vi "7903 Port 5 Constructor.vi"(11 "aurora instance (0)":u8) -> (3 "aurora64b66b buffered":refnum<class "Aurora64b66b Buffered.lvclass">)   [LabVIEW 2023, in "PXIe-7903 Aurora Example.lvlib"]
uses:
  PXIe-7903 Aurora Example.lvlib
  Program Files/NI/LVAddons/niidl/1/instr.lib/_niInstr/Aurora64b66b/v1/Shared/Buffered/Link Mode.ctl
  Program Files/NI/LVAddons/niidl/1/instr.lib/_niInstr/Aurora64b66b/v1/Shared/niInstr Aurora64b66b v1 Shared.lvlib
  Program Files/NI/LVAddons/niidl/1/instr.lib/_niInstr/Aurora64b66b/v1/Shared/Basic/Endianness.ctl
  Program Files/NI/LVAddons/niidl/1/instr.lib/_niInstr/Aurora64b66b/v1/Shared/Basic/GT Type.ctl
  Program Files/NI/LVAddons/niidl/1/instr.lib/_niInstr/Aurora64b66b/v1/Shared/Basic/Aurora Config.ctl
  Program Files/NI/LVAddons/niidl/1/instr.lib/_niInstr/CLIP Adapters/v1/FPGA/AXI4-Lite/FXP32 Address - FXP32 Data/Public/CLIP Resources.ctl
  Program Files/NI/LVAddons/niidl/1/instr.lib/_niInstr/CLIP Adapters/v1/FPGA/AXI4-Lite/FXP32 Address - FXP32 Data/niInstr AXI4-Lite - FXP32 Address - FXP32 Data v1 FPGA.lvclass
  Program Files/NI/LVAddons/niidl/1/instr.lib/_niInstr/Aurora64b66b/v1/FPGA/Basic/Public/TypeDefs/CLIP Parameters.ctl
  Program Files/NI/LVAddons/niidl/1/instr.lib/_niInstr/Aurora64b66b/v1/FPGA/Basic/Aurora64b66b Basic.lvclass
  Program Files/NI/LVAddons/niidl/1/instr.lib/_niInstr/Aurora64b66b/v1/FPGA/Buffered/Aurora64b66b Buffered.lvclass
  Program Files/NI/LVAddons/niidl/1/instr.lib/_niInstr/Aurora64b66b/v1/FPGA/Basic/Public/TypeDefs/Tx Data CLIP IO.ctl
  Program Files/NI/LVAddons/niidl/1/instr.lib/_niInstr/Aurora64b66b/v1/FPGA/Basic/Public/TypeDefs/Rx Data CLIP IO.ctl
  Program Files/NI/LVAddons/niidl/1/instr.lib/_niInstr/Aurora64b66b/v1/FPGA/Basic/Public/TypeDefs/NFC CLIP IO.ctl
  Program Files/NI/LVAddons/niidl/1/instr.lib/_niInstr/Aurora64b66b/v1/FPGA/Basic/Public/TypeDefs/Link Status CLIP IO.ctl
  Program Files/NI/LVAddons/niidl/1/instr.lib/_niInstr/Aurora64b66b/v1/FPGA/Basic/Public/TypeDefs/Reset CLIP IO.ctl
  Program Files/NI/LVAddons/niidl/1/instr.lib/_niInstr/Aurora64b66b/v1/FPGA/Basic/Public/TypeDefs/CRC CLIP IO.ctl
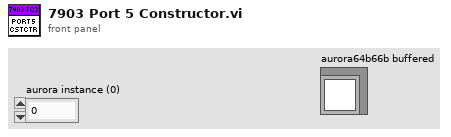
[diagram p1: front panel]
types:
  T1 = typedef "niInstr Aurora64b66b v1 FPGA.lvlib/Aurora64b66b Basic.lvclass/CLIP Parameters.ctl" = cluster{"crc clip io":T2, "reset clip io":T3, "link status clip io":T4, "nfc clip io":T5, "user clock":refnum<k21>, "rx data ":T6, "tx data":T7, "axi drp clip resources":T8, "axi control clip resources":T8}
  T2 = typedef "niInstr Aurora64b66b v1 FPGA.lvlib/Aurora64b66b Basic.lvclass/CRC CLIP IO.ctl" = cluster{"crc pass fail n":refnum<k21>, "crc valid":refnum<k21>}
  T3 = typedef "niInstr Aurora64b66b v1 FPGA.lvlib/Aurora64b66b Basic.lvclass/Reset CLIP IO.ctl" = cluster{"reset pb":refnum<k21>, "pma init":refnum<k21>, "link reset":refnum<k21>}
  T4 = typedef "niInstr Aurora64b66b v1 FPGA.lvlib/Aurora64b66b Basic.lvclass/Link Status CLIP IO.ctl" = cluster{"hard error":refnum<k21>, "soft error":refnum<k21>, "lane up 8":refnum<k21>, "channel up":refnum<k21>, "sys reset":refnum<k21>, "mmcm not locked":refnum<k21>, "lane up 4":refnum<k21>}
  T5 = typedef "niInstr Aurora64b66b v1 FPGA.lvlib/Aurora64b66b Basic.lvclass/NFC CLIP IO.ctl" = cluster{"s_axis_tvalid":refnum<k21>, "s_axis_tdata":refnum<k21>, "s_axis_tready":refnum<k21>}
  T6 = typedef "niInstr Aurora64b66b v1 FPGA.lvlib/Aurora64b66b Basic.lvclass/Rx Data CLIP IO.ctl" = cluster{"m_axis_tvalid":refnum<k21>, "m_axis_tdata0":refnum<k21>, "m_axis_tdata1":refnum<k21>, "m_axis_tdata 2":refnum<k21>, "m_axis_tdata 3":refnum<k21>, "m_axis_tdata4":refnum<k21>, "m_axis_tdata5":refnum<k21>, "m_axis_tdata6":refnum<k21>, "m_axis_tdata7":refnum<k21>, "m_axis_tlast":refnum<k21>, "m_axis_tkeep1":refnum<k21>, "m_axis_tkeep2":refnum<k21>, "m_axis_tkeep4":refnum<k21>, "m_axis_tkeep8":refnum<k21>}
  T7 = typedef "niInstr Aurora64b66b v1 FPGA.lvlib/Aurora64b66b Basic.lvclass/Tx Data CLIP IO.ctl" = cluster{"s_axis_tvalid":refnum<k21>, "s_axis_tdata0":refnum<k21>, "s_axis_tdata1":refnum<k21>, "s_axis_tdata2":refnum<k21>, "s_axis_tdata3":refnum<k21>, "s_axis_tdata4":refnum<k21>, "s_axis_tdata5":refnum<k21>, "s_axis_tdata6":refnum<k21>, "s_axis_tdata7":refnum<k21>, "s_axis_tready":refnum<k21>, "s_axis_tlast":refnum<k21>, "s_axis_tkeep":refnum<k21>}
  T8 = typedef "niInstr AXI4-Lite - FXP32 Address - FXP32 Data v1 FPGA.lvclass/CLIP Resources.ctl" = cluster{"s_axi_araddr":refnum<k21>, "s_axi_arvalid":refnum<k21>, "s_axi_arready":refnum<k21>, "s_axi_rdata":refnum<k21>, "s_axi_rresp":refnum<k21>, "s_axi_rvalid":refnum<k21>, "s_axi_rready":refnum<k21>, "s_axi_awaddr":refnum<k21>, "s_axi_awvalid":refnum<k21>, "s_axi_awready":refnum<k21>, "s_axi_wdata":refnum<k21>, "s_axi_wstrb":refnum<k21>, "s_axi_wvalid":refnum<k21>, "s_axi_wready":refnum<k21>, "s_axi_bresp":refnum<k21>, "s_axi_bvalid":refnum<k21>, "s_axi_bready":refnum<k21>}
  T9 = typedef "niInstr Aurora64b66b v1 Shared.lvlib/Endianness.ctl" = enum16{"little", "big"}
  T10 = typedef "niInstr Aurora64b66b v1 Shared.lvlib/GT Type.ctl" = enum16{"gtxe2", "gthe2", "gthe3", "gtye4"}
  T11 = typedef "niInstr Aurora64b66b v1 Shared.lvlib/Aurora Config.ctl" = cluster{"packets enabled":bool, "nfc immediate enabled":bool, "crc enabled":bool, "ref clk frequency":u64, "line rate":u64, "port number":u8, "number of lanes":u8, "reference clock index":u8, "gt type":T10, "endianness":T9}
  T12 = typedef "niInstr Aurora64b66b v1 Shared.lvlib/Link Mode.ctl" = enum16{"duplex", "tx only", "rx only"}
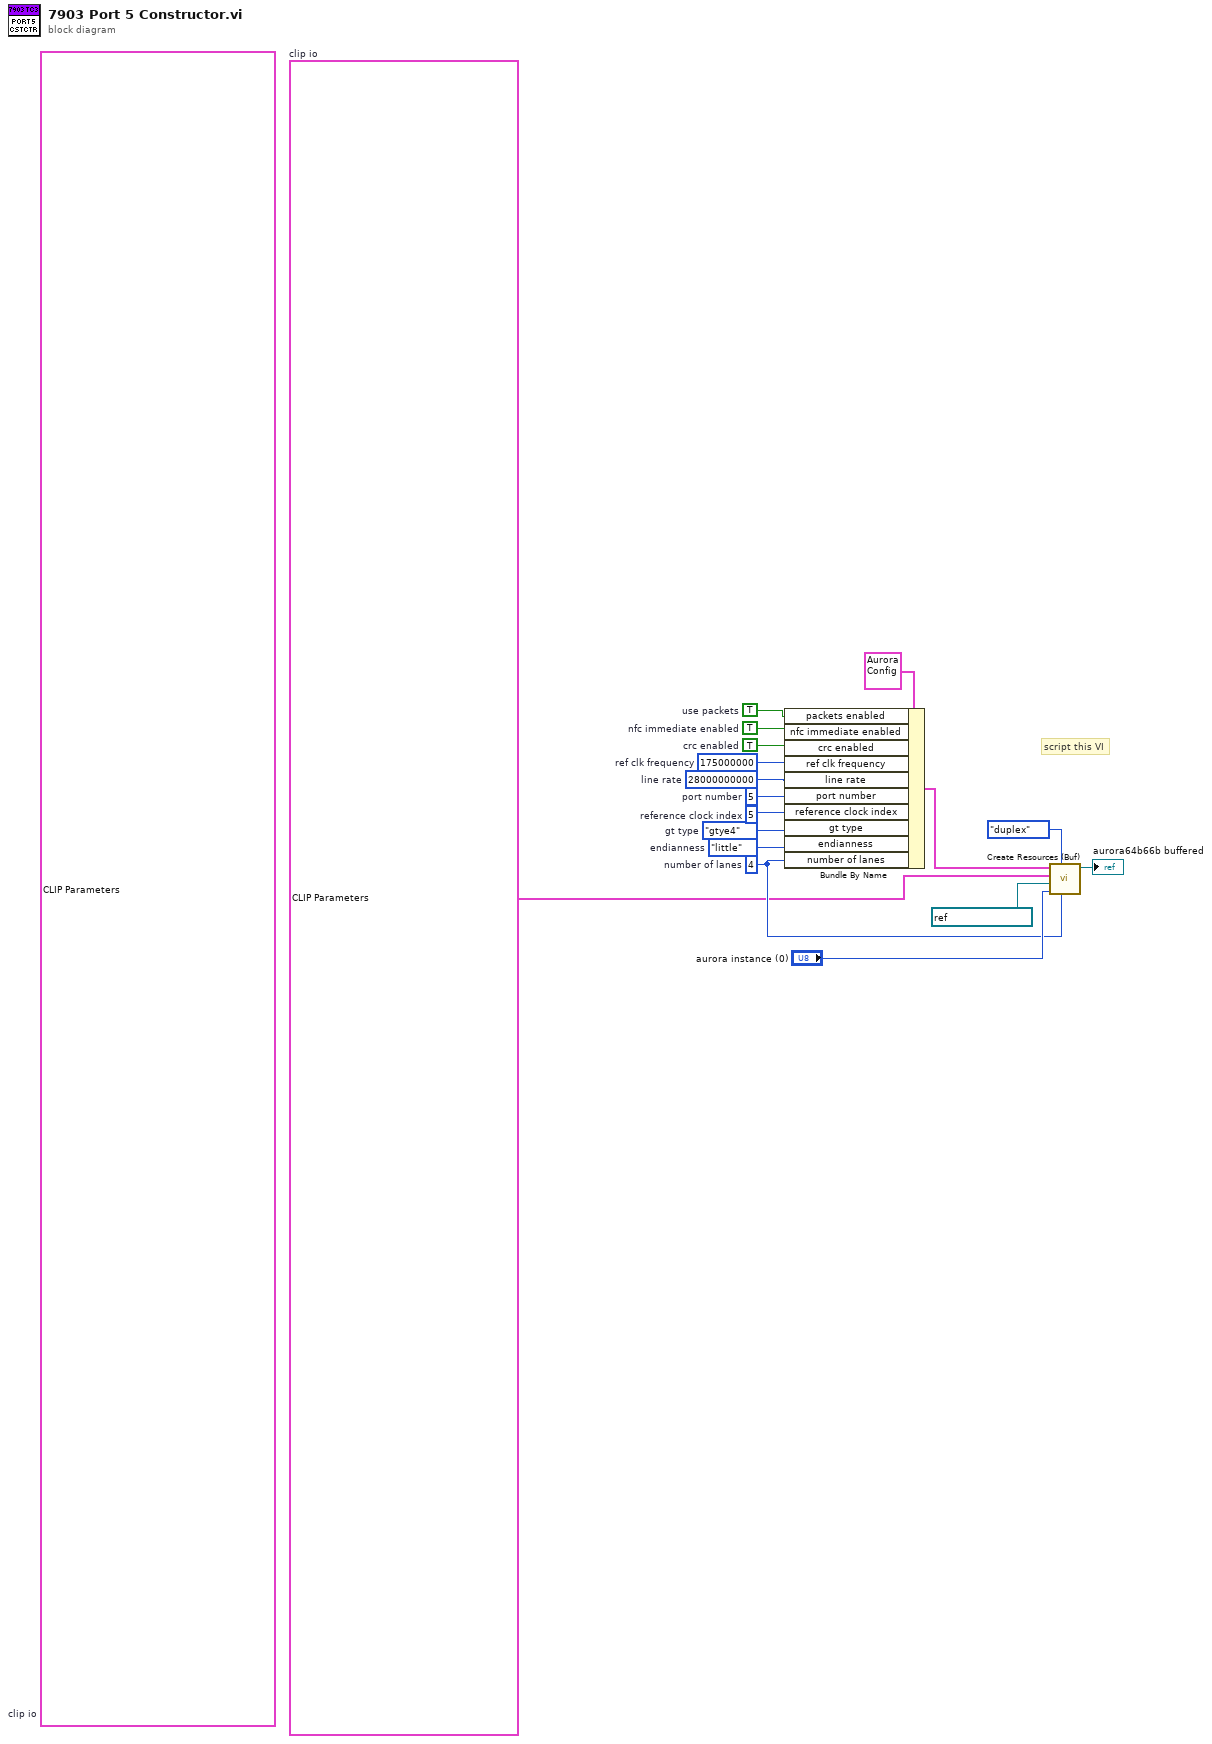
[diagram p0: block diagram]
diagram:
  w1 = T1 {"crc clip io"={"crc pass fail n"="IO Socket.Port5.CrcPassFail_n", "crc valid"="IO Socket.Port5.CrcValid"}, "reset clip io"={"reset pb"="IO Socket.Port5.ResetPb", "pma init"="IO Socket.Port5.PmaInit", "link reset"="IO Socket.Port5.LinkResetOut"}, "link status clip io"={"hard error"="IO Socket.Port5.HardError", "soft error"="IO Socket.Port5.SoftError", "lane up 8"="IO Socket.Port5.LaneUp", "channel up"="IO Socket.Port5.ChannelUp", "sys reset"="IO Socket.Port5.SysResetOut", "mmcm not locked"="IO Socket.Port5.MmcmNotLockOut", "lane up 4"="IO Socket.Port5.LaneUp"}, "nfc clip io"={"s_axis_tvalid"="IO Socket.Port5.Nfc.TValid", "s_axis_tdata"="IO Socket.Port5.Nfc.TData", "s_axis_tready"="IO Socket.Port5.Nfc.TReady"}, "user clock"="IO Socket.Port5 User Clock", "rx data "={"m_axis_tvalid"="IO Socket.Port5.Rx.TValid", "m_axis_tdata0"="IO Socket.Port5.Rx.TData0", "m_axis_tdata1"="IO Socket.Port5.Rx.TData1", "m_axis_tdata 2"="IO Socket.Port5.Rx.TData2", "m_axis_tdata 3"="IO Socket.Port5.Rx.TData3", "m_axis_tdata4"="IO Socket.Port5.Rx.TData4", "m_axis_tdata5"="IO Socket.Port5.Rx.TData5", "m_axis_tdata6"="IO Socket.Port5.Rx.TData6", "m_axis_tdata7"="IO Socket.Port5.Rx.TData7", "m_axis_tlast"="IO Socket.Port5.Rx.TLast", "m_axis_tkeep1"="IO Socket.Port5.Rx.TKeep", "m_axis_tkeep2"="IO Socket.Port5.Rx.TKeep", "m_axis_tkeep4"="IO Socket.Port5.Rx.TKeep", "m_axis_tkeep8"="IO Socket.Port5.Rx.TKeep"}, "tx data"={"s_axis_tvalid"="IO Socket.Port5.Tx.TValid", "s_axis_tdata0"="IO Socket.Port5.Tx.TData0", "s_axis_tdata1"="IO Socket.Port5.Tx.TData1", "s_axis_tdata2"="IO Socket.Port5.Tx.TData2", "s_axis_tdata3"="IO Socket.Port5.Tx.TData3", "s_axis_tdata4"="IO Socket.Port5.Tx.TData4", "s_axis_tdata5"="IO Socket.Port5.Tx.TData5", "s_axis_tdata6"="IO Socket.Port5.Tx.TData6", "s_axis_tdata7"="IO Socket.Port5.Tx.TData7", "s_axis_tready"="IO Socket.Port5.Tx.TReady", "s_axis_tlast"="IO Socket.Port5.Tx.TLast", "s_axis_tkeep"="IO Socket.Port5.Tx.TKeep"}, "axi drp clip resources"={"s_axi_araddr"="IO Socket.Port5.DrpChAxi.ARAddr", "s_axi_arvalid"="IO Socket.Port5.DrpChAxi.ARValid", "s_axi_arready"="IO Socket.Port5.DrpChAxi.ARReady", "s_axi_rdata"="IO Socket.Port5.DrpChAxi.RData", "s_axi_rresp"="IO Socket.Port5.DrpChAxi.RResp", "s_axi_rvalid"="IO Socket.Port5.DrpChAxi.RValid", "s_axi_rready"="IO Socket.Port5.DrpChAxi.RReady", "s_axi_awaddr"="IO Socket.Port5.DrpChAxi.AWAddr", "s_axi_awvalid"="IO Socket.Port5.DrpChAxi.AWValid", "s_axi_awready"="IO Socket.Port5.DrpChAxi.AWReady", "s_axi_wdata"="IO Socket.Port5.DrpChAxi.WData", "s_axi_wstrb"="IO Socket.Port5.DrpChAxi.WStrb", "s_axi_wvalid"="IO Socket.Port5.DrpChAxi.WValid", "s_axi_wready"="IO Socket.Port5.DrpChAxi.WReady", "s_axi_bresp"="IO Socket.Port5.DrpChAxi.BResp", "s_axi_bvalid"="IO Socket.Port5.DrpChAxi.BValid", "s_axi_bready"="IO Socket.Port5.DrpChAxi.BReady"}, "axi control clip resources"={"s_axi_araddr"="IO Socket.Port5.CtrlAxi.ARAddr", "s_axi_arvalid"="IO Socket.Port5.CtrlAxi.ARValid", "s_axi_arready"="IO Socket.Port5.CtrlAxi.ARReady", "s_axi_rdata"="IO Socket.Port5.CtrlAxi.RData", "s_axi_rresp"="IO Socket.Port5.CtrlAxi.RResp", "s_axi_rvalid"="IO Socket.Port5.CtrlAxi.RValid", "s_axi_rready"="IO Socket.Port5.CtrlAxi.RReady", "s_axi_awaddr"="IO Socket.Port5.CtrlAxi.AWAddr", "s_axi_awvalid"="IO Socket.Port5.CtrlAxi.AWValid", "s_axi_awready"="IO Socket.Port5.CtrlAxi.AWReady", "s_axi_wdata"="IO Socket.Port5.CtrlAxi.WData", "s_axi_wstrb"="IO Socket.Port5.CtrlAxi.WStrb", "s_axi_wvalid"="IO Socket.Port5.CtrlAxi.WValid", "s_axi_wready"="IO Socket.Port5.CtrlAxi.WReady", "s_axi_bresp"="IO Socket.Port5.CtrlAxi.BResp", "s_axi_bvalid"="IO Socket.Port5.CtrlAxi.BValid", "s_axi_bready"="IO Socket.Port5.CtrlAxi.BReady"}}  # clip io
  (unwired) T1 {"crc clip io"={"crc pass fail n"="IO Socket\\Port5\\CrcPassFail_n", "crc valid"="IO Socket\\Port5\\CrcValid"}, "reset clip io"={"reset pb"="IO Socket\\Port5\\ResetPb", "pma init"="IO Socket\\Port5\\PmaInit", "link reset"="IO Socket\\Port5\\LinkResetOut"}, "link status clip io"={"hard error"="IO Socket\\Port5\\HardError", "soft error"="IO Socket\\Port5\\SoftError", "lane up 8"="IO Socket\\Port5\\LaneUp", "channel up"="IO Socket\\Port5\\ChannelUp", "sys reset"="IO Socket\\Port5\\SysResetOut", "mmcm not locked"="IO Socket\\Port5\\MmcmNotLockOut", "lane up 4"="IO Socket\\Port5\\LaneUp"}, "nfc clip io"={"s_axis_tvalid"="IO Socket\\Port5\\Nfc\\TValid", "s_axis_tdata"="IO Socket\\Port5\\Nfc\\TData", "s_axis_tready"="IO Socket\\Port5\\Nfc\\TReady"}, "user clock"="IO Socket.Port5 User Clock", "rx data "={"m_axis_tvalid"="IO Socket\\Port5\\Rx\\TValid", "m_axis_tdata0"="IO Socket\\Port5\\Rx\\TData0", "m_axis_tdata1"="IO Socket\\Port5\\Rx\\TData1", "m_axis_tdata 2"="IO Socket\\Port5\\Rx\\TData2", "m_axis_tdata 3"="IO Socket\\Port5\\Rx\\TData3", "m_axis_tdata4"="IO Socket\\Port5\\Rx\\TData4", "m_axis_tdata5"="IO Socket\\Port5\\Rx\\TData5", "m_axis_tdata6"="IO Socket\\Port5\\Rx\\TData6", "m_axis_tdata7"="IO Socket\\Port5\\Rx\\TData7", "m_axis_tlast"="IO Socket\\Port5\\Rx\\TLast", "m_axis_tkeep1"="IO Socket\\Port5\\Rx\\TKeep", "m_axis_tkeep2"="IO Socket\\Port5\\Rx\\TKeep", "m_axis_tkeep4"="IO Socket\\Port5\\Rx\\TKeep", "m_axis_tkeep8"="IO Socket\\Port5\\Rx\\TKeep"}, "tx data"={"s_axis_tvalid"="IO Socket\\Port5\\Tx\\TValid", "s_axis_tdata0"="IO Socket\\Port5\\Tx\\TData0", "s_axis_tdata1"="IO Socket\\Port5\\Tx\\TData1", "s_axis_tdata2"="IO Socket\\Port5\\Tx\\TData2", "s_axis_tdata3"="IO Socket\\Port5\\Tx\\TData3", "s_axis_tdata4"="IO Socket\\Port5\\Tx\\TData4", "s_axis_tdata5"="IO Socket\\Port5\\Tx\\TData5", "s_axis_tdata6"="IO Socket\\Port5\\Tx\\TData6", "s_axis_tdata7"="IO Socket\\Port5\\Tx\\TData7", "s_axis_tready"="IO Socket\\Port5\\Tx\\TReady", "s_axis_tlast"="IO Socket\\Port5\\Tx\\TLast", "s_axis_tkeep"="IO Socket\\Port5\\Tx\\TKeep"}, "axi drp clip resources"={"s_axi_araddr"="IO Socket\\Port5\\DrpChAxi\\ARAddr", "s_axi_arvalid"="IO Socket\\Port5\\DrpChAxi\\ARValid", "s_axi_arready"="IO Socket\\Port5\\DrpChAxi\\ARReady", "s_axi_rdata"="IO Socket\\Port5\\DrpChAxi\\RData", "s_axi_rresp"="IO Socket\\Port5\\DrpChAxi\\RResp", "s_axi_rvalid"="IO Socket\\Port5\\DrpChAxi\\RValid", "s_axi_rready"="IO Socket\\Port5\\DrpChAxi\\RReady", "s_axi_awaddr"="IO Socket\\Port5\\DrpChAxi\\AWAddr", "s_axi_awvalid"="IO Socket\\Port5\\DrpChAxi\\AWValid", "s_axi_awready"="IO Socket\\Port5\\DrpChAxi\\AWReady", "s_axi_wdata"="IO Socket\\Port5\\DrpChAxi\\WData", "s_axi_wstrb"="IO Socket\\Port5\\DrpChAxi\\WStrb", "s_axi_wvalid"="IO Socket\\Port5\\DrpChAxi\\WValid", "s_axi_wready"="IO Socket\\Port5\\DrpChAxi\\WReady", "s_axi_bresp"="IO Socket\\Port5\\DrpChAxi\\BResp", "s_axi_bvalid"="IO Socket\\Port5\\DrpChAxi\\BValid", "s_axi_bready"="IO Socket\\Port5\\DrpChAxi\\BReady"}, "axi control clip resources"={"s_axi_araddr"="IO Socket\\Port5\\CtrlAxi\\ARAddr", "s_axi_arvalid"="IO Socket\\Port5\\CtrlAxi\\ARValid", "s_axi_arready"="IO Socket\\Port5\\CtrlAxi\\ARReady", "s_axi_rdata"="IO Socket\\Port5\\CtrlAxi\\RData", "s_axi_rresp"="IO Socket\\Port5\\CtrlAxi\\RResp", "s_axi_rvalid"="IO Socket\\Port5\\CtrlAxi\\RValid", "s_axi_rready"="IO Socket\\Port5\\CtrlAxi\\RReady", "s_axi_awaddr"="IO Socket\\Port5\\CtrlAxi\\AWAddr", "s_axi_awvalid"="IO Socket\\Port5\\CtrlAxi\\AWValid", "s_axi_awready"="IO Socket\\Port5\\CtrlAxi\\AWReady", "s_axi_wdata"="IO Socket\\Port5\\CtrlAxi\\WData", "s_axi_wstrb"="IO Socket\\Port5\\CtrlAxi\\WStrb", "s_axi_wvalid"="IO Socket\\Port5\\CtrlAxi\\WValid", "s_axi_wready"="IO Socket\\Port5\\CtrlAxi\\WReady", "s_axi_bresp"="IO Socket\\Port5\\CtrlAxi\\BResp", "s_axi_bvalid"="IO Socket\\Port5\\CtrlAxi\\BValid", "s_axi_bready"="IO Socket\\Port5\\CtrlAxi\\BReady"}}  # clip io
  w4 = u8 4  # number of lanes
  w6 = Endianness."little"  # endianness
  w7 = GT_Type."gtye4"  # gt type
  w8 = u8 5  # port number
  w9 = u64 28000000000  # line rate
  w10 = u64 175000000  # ref clk frequency
  w11 = TRUE  # crc enabled
  w12 = TRUE  # nfc immediate enabled
  w13 = TRUE  # use packets
  w14 = u8 5  # reference clock index
  # "script this VI"
  n1 = Bundle By Name(cluster=T11 {"packets enabled"=TRUE, "nfc immediate enabled"=TRUE, "crc enabled"=TRUE, "ref clk frequency"=312501000, "line rate"=10416700000, "port number"=1, "number of lanes"=4, "reference clock index"=0, "gt type"=enum."gtye4", "endianness"=enum."little"} ("aurora port config"), "packets enabled"=w13, "nfc immediate enabled"=w12, "crc enabled"=w11, "ref clk frequency"=w10, "line rate"=w9, "port number"=w8, "reference clock index"=w14, "gt type"=w7, "endianness"=w6, "number of lanes"=w4) -> (w5:T11)
  n2 = call "Create Resources (Buf).vi"("number of lanes"=w4, "link mode"=Link_Mode."duplex", "instance (0)"="aurora instance (0)", "init clk"=refnum<k21> "80 MHz Clock", "clip io"=w1, "aurora port config"=w5) -> ("aurora64b66b buffered"=→"aurora64b66b buffered":refnum<class "Aurora64b66b Buffered.lvclass">)  [unwired: 5 in]
